vi "ACT_6_Task1_825005609.vi"() -> ()   [LabVIEW 2016]
panel:
  out "Divide":i32
  out "Multiply":dbl
  out "Subtract":dbl
  out "Addition":dbl
  in  "Numeric 2":dbl
  in  "Numeric":dbl
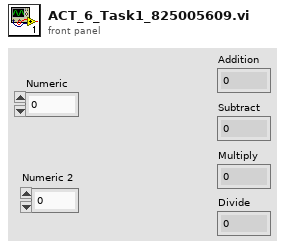
[diagram p1: front panel]
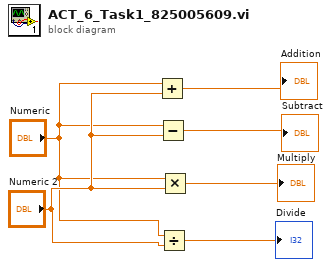
[diagram p0: block diagram]
diagram:
  n1 = Add(x="Numeric", y="Numeric 2") -> (x+y=→"Addition":dbl)
  n2 = Subtract(x="Numeric", y="Numeric 2") -> (x-y=→"Subtract":dbl)
  n3 = Divide(x="Numeric", y="Numeric 2") -> (x/y=→"Divide":dbl)
  n4 = Multiply(x="Numeric", y="Numeric 2") -> (x*y=→"Multiply":dbl)
